vi "10 Tap 8-Bit.vi"() -> (0 "Pixels":T1)   [LabVIEW 2013]
uses:
  <vilib>/rvi/eio/common/nirviEmuTemplateMethod_errors.vi
  <vilib>/eio/EIONode/EIONode.xnode
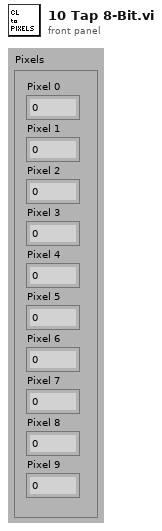
[diagram p1: front panel]
types:
  T1 = cluster{"Pixel 0":u8, "Pixel 1":u8, "Pixel 2":u8, "Pixel 3":u8, "Pixel 4":u8, "Pixel 5":u8, "Pixel 6":u8, "Pixel 7":u8, "Pixel 8":u8, "Pixel 9":u8}
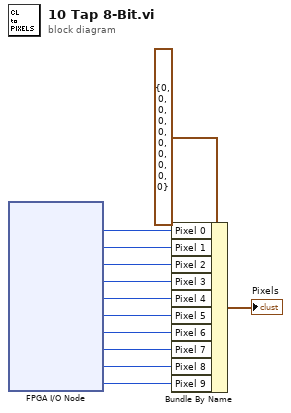
[diagram p0: block diagram]
diagram:
  n1 = xnode "FPGA I/O Node"() -> ("CL Port A"=w12:u8, "CL Port B"=w11:u8, "CL Port C"=w10:u8, "CL Port D"=w9:u8, "CL Port E"=w8:u8, "CL Port F"=w7:u8, "CL Port G"=w6:u8, "CL Port H"=w5:u8, "CL Port I"=w3:u8, "CL Port J"=w2:u8)  [unwired: 10 in, 10 out]
  n2 = Bundle By Name(cluster=T1 {"Pixel 0"=0, "Pixel 1"=0, "Pixel 2"=0, "Pixel 3"=0, "Pixel 4"=0, "Pixel 5"=0, "Pixel 6"=0, "Pixel 7"=0, "Pixel 8"=0, "Pixel 9"=0} ("PixelData"), "Pixel 0"=w12, "Pixel 1"=w11, "Pixel 2"=w10, "Pixel 3"=w9, "Pixel 4"=w8, "Pixel 5"=w7, "Pixel 6"=w6, "Pixel 7"=w5, "Pixel 8"=w3, "Pixel 9"=w2) -> (→"Pixels":T1)
